vi "Add Trigger to Acyclic Frames Section.vi"(8 "error in":errorcluster, 10 "trigger name":string, 11 "acyclic frames section":T1 format="%.0x") -> (0 "error out":errorcluster, 2 "acyclic frame trigger":T1 format="%.0x", 3 "acyclic frames section out":T1 format="%.0x")   [LabVIEW 2020, in "AIM MIL-STD-1553 Scripting.lvlib"]
doc: "Adds an <b>acyclic frame trigger</b> to the specified <b>acyclic frames section</b>. Uses the specified <b>trigger name</b> (if trigger name is an empty string, uses the default value)."
uses:
  AIM MIL-STD-1553 Scripting.lvlib
  <vilib>/NI VeriStand/Custom Device API/Custom Device Item Ref.ctl
  <vilib>/NI VeriStand/Custom Device API/Custom Device Channel.ctl
  <vilib>/NI VeriStand/Custom Device API/Custom Device Channel Type.ctl
  Constants.vi
  <vilib>/NI VeriStand/Custom Device API/Custom Device API.lvlib
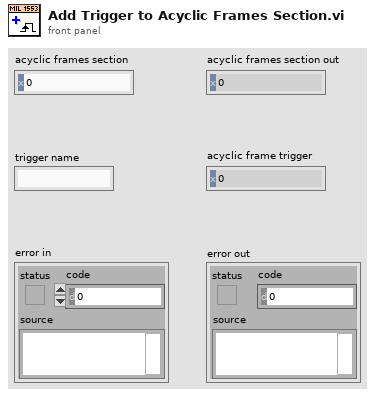
[diagram p1: front panel]
types:
  T1 = typedef "Custom Device API.lvlib/Custom Device Item Ref.ctl" = u64
  T2 = typedef "Custom Device API.lvlib/Custom Device Channel.ctl" = cluster{"Type":T3, "Units":string, "Default Value":dbl, "Faultable":bool, "Scalable":bool}
  T3 = typedef "Custom Device API.lvlib/Custom Device Channel Type.ctl" = enum16{"Input", "Output"}
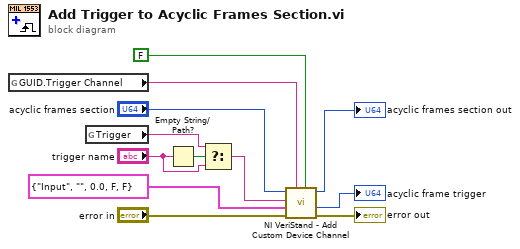
[diagram p0: block diagram]
diagram:
  n1 = global read "Constants.vi" "GUID.Trigger Channel"() -> (w2:string)
  n2 = global read "Constants.vi" "Trigger"() -> (w4:string)
  n3 = Empty String/Path?(string/path="trigger name") -> (empty?=w6:bool)
  n4 = Select(t=w4, s=w6, f="trigger name") -> (s? t:f=w3:string)
  n5 = call <vilib>:"NI VeriStand - Add Custom Device Channel.vi"("Highlight? (F)"=FALSE, "GUID (Default Channel)"=w2, "error in (no error)"="error in", "Channel"=T2 {"Type"=enum."Input", "Units"="", "Default Value"=0.0, "Faultable"=FALSE, "Scalable"=FALSE}, "Channel Name"=w3, "Parent Ref in"="acyclic frames section") -> ("error out"=→"error out":errorcluster, "Channel Ref"=→"acyclic frame trigger":T1, "Parent Ref out"=→"acyclic frames section out":T1)  [unwired: 2 in, 1 out]
